vi "Acquire.vi"(8 "error in (no error)":errorcluster, 10 "Message Queues":T1, 11 "Hardware Resources in":T4) -> (0 "error out":errorcluster, 2 "Message Queues out":T1, 3 "Hardware Resources out":T4)   [LabVIEW 2018, in "Acquisition.lvlib"]
doc: "Perform the acquisition. Replace the contents of this diagram with calls to acquisition hardware."
uses:
  Acquisition.lvlib
  Hardware Configuration.ctl
  Signal Type.ctl
  Support/Message Queue/All Message Queues.ctl
  Support/Message Queue/Message Cluster.ctl
  Controls/Data Queue.ctl
  library/Datalogger LLB/Data Record Control.ctl
  Controls/Data Notifier.ctl
  support/Message Queue/Message Queue.lvlib
  library/Datalogger LLB/Datalogger.lvclass
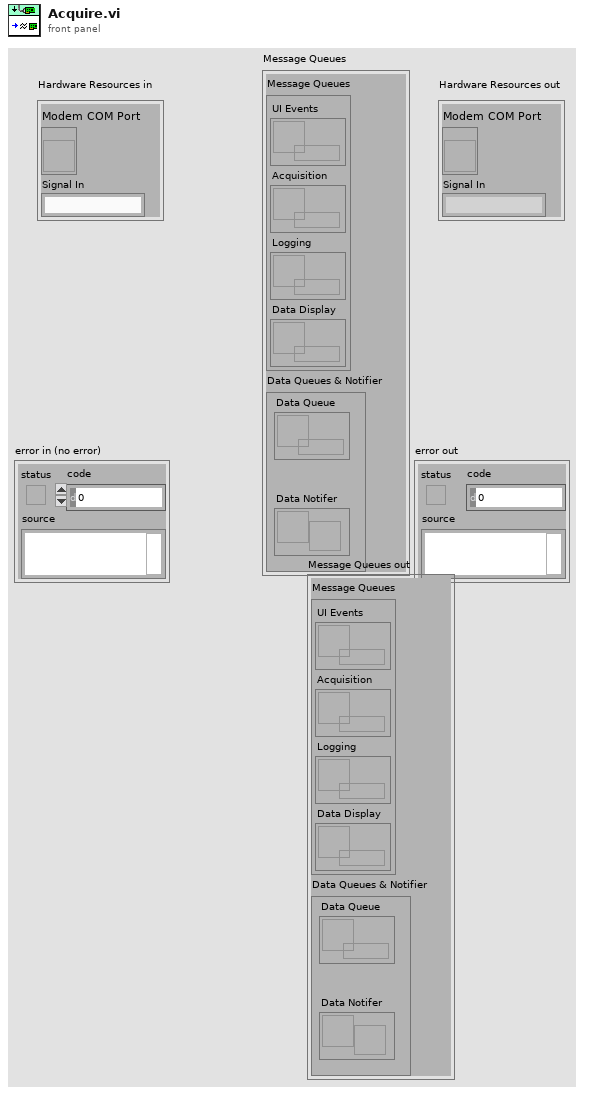
[diagram p1: front panel]
types:
  T1 = typedef "Message Queue.lvlib/All Message Queues.ctl" = cluster{"Message Queues":cluster{"UI Events":refnum<queue>, "Acquisition":refnum<queue>, "Logging":refnum<queue>, "Data Display":refnum<queue>}, "Data Queues & Notifier":cluster{"Data Queue":T2, "Data Notifer":T3}}
  T2 = typedef "Data Queue.ctl" = refnum<queue>
  T3 = typedef "Data Notifier.ctl" = refnum<notifier>
  T4 = typedef "Acquisition.lvlib/Hardware Configuration.ctl" = cluster{"Modem COM Port":refnum<vi>, "Signal In":T5}
  T5 = typedef "Acquisition.lvlib/Signal Type.ctl" = string
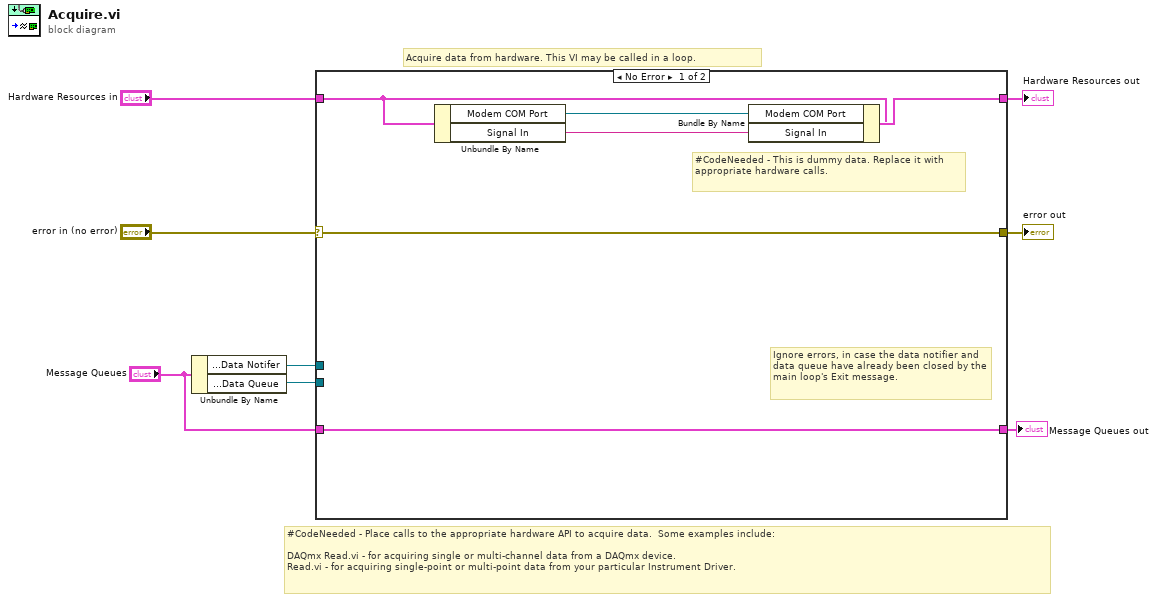
[diagram p0: block diagram]
diagram:
  # "Acquire data from hardware. This VI may be called in a loop."
  # "#CodeNeeded - Place calls to the appropriate hardware API to acquire data.  Some examples include:\n\nDAQmx Read.vi - for acquiring single or multi-channel data from a DAQmx device.\nRead.vi - for acquiring single-point or multi-point data from your particular Instrument Driver."
  n1 = Unbundle By Name("Message Queues") -> ("Data Queues & Notifier.Data Notifer"=w4:T3, "Data Queues & Notifier.Data Queue"=w3:T2)
  n2 = case shown="No Error" "error in (no error)" {
    selector: "error in (no error)" -> [w13 w16]
    tunnel: [w13 w16] -> w7
    tunnel: "Hardware Resources in" -> [w10 w17]
    tunnel: [w14 w17] -> w5
    tunnel: w4 -> [_ _]
    tunnel: w3 -> [_ _]
    tunnel: "Message Queues" -> [w9 w15]
    tunnel: [w9 w15] -> w1
    frame No Error {
      # "Ignore errors, in case the data notifier and data queue have already been closed by the main loop's Exit message."
      # "#CodeNeeded - This is dummy data. Replace it with appropriate hardware calls."
      n3 = Unbundle By Name(w10) -> ("Modem COM Port"=w11:refnum<vi>, "Signal In"=w12:T5)
      n4 = Bundle By Name(cluster=w10, "Modem COM Port"=w11, "Signal In"=w12) -> (w14:T4)
    }
    frame Error {
    }
  }
  "Hardware Resources out" <- w5
  "error out" <- w7
  "Message Queues out" <- w1
